vi "Do Task.vi"(8 "error in":errorcluster, 9 "Task Ident":string, 10 "Input":variant, 11 "Series Actor in":refnum<class "Series Actor.lvclass">) -> (0 "error out":errorcluster, 3 "Series Actor out":refnum<class "Series Actor.lvclass">)   [LabVIEW 2023, in "Series Actor.lvlib" / "Series Actor.lvclass"]
uses:
  Series Actor.lvclass
  Series Actor.lvclass/Series Actor.ctl
  Task/ITask Actor/ITask Actor Messages/Do Msg/Do Msg.lvclass/Do Msg.ctl
  <vilib>/ActorFramework/Message Enqueuer/Message Enqueuer.lvclass/Message Enqueuer.ctl
  <vilib>/ActorFramework/Message Enqueuer/Enqueue.vi
  Task/ITask Actor/ITask Actor Messages/Do Msg/Do Msg.lvclass
  C:/Program Files/National Instruments/LabVIEW 2023/vi.lib/ActorFramework/Message/Message.lvclass
  <vilib>/Utility/error.llb/Error Cluster From Error Code.vi
  <vilib>/Utility/LVClass/Get LV Class Name.vi
  <resource>/AFDebug/Generate Trace for Message.vi
  <vilib>/ActorFramework/Message Priority Queue/Priority Enqueue.vi
  <vilib>/ErrorRing/Error Ring.xnode
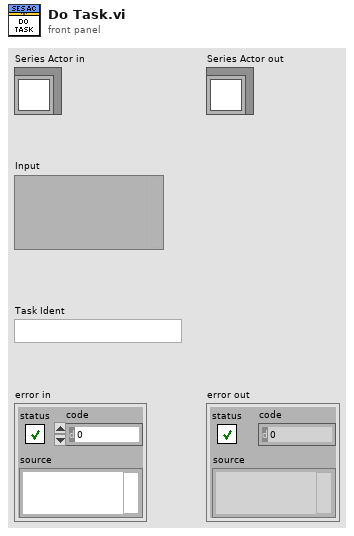
[diagram p1: front panel]
types:
  T1 = map{string, refnum<class "Message Enqueuer.lvclass">}
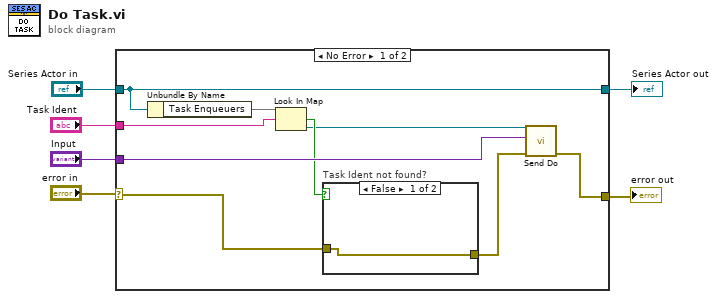
[diagram p0: block diagram]
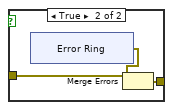
[diagram p2: hidden frame]
diagram:
  n1 = case shown="No Error" "error in" {
    selector: "error in" -> [w9 w26]
    tunnel: "Series Actor in" -> [w14 w25]
    tunnel: [w14 w25] -> w5
    tunnel: [w15 w26] -> w1
    tunnel: "Task Ident" -> [w12 _]
    tunnel: "Input" -> [w11 _]
    frame No Error {
      n2 = Unbundle By Name(w14) -> ("Task Enqueuers"=w13:T1)
      n3 = Look In Map(map=w13, key=w12) -> (key not found?=w10:bool, value=w7:refnum<class "Message Enqueuer.lvclass">)  [unwired: 1 in]
      n4 = case "Task Ident not found?" shown="False" w10 {
        tunnel: w9 -> [w16 w19]
        tunnel: [w16 w17] -> w8
        frame False {
        }
        frame True {
          n5 = xnode "Error Ring"() -> ("error out"=w18:errorcluster)
          n6 = Merge Errors(w19, w18) -> (w17:errorcluster)
        }
      }
      n7 = call "Send Do.vi"("error in (no error)"=w8, "Input"=w11, "Message Enqueuer"=w7) -> ("error out"=w15:errorcluster)  [unwired: 7 in, 1 out]
    }
    frame Error {
    }
  }
  "error out" <- w1
  "Series Actor out" <- w5
